vi "VISA停止_G.vi"() -> ()   [LabVIEW 2021]
panel:
  out "VISA停止_\nグローバル":bool
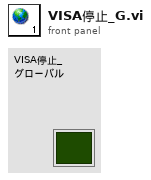
[diagram p1: front panel]
diagram:
